vi "update-table-data.vi"(8 "error in (no error)":errorcluster, 9 "valid":bool, 10 "CAN frame":T1 {"payload" format="%x"; "timestamp" format="%<%.7X\n%x>T"; "type" items=["CAN Data"=0, "CAN Remote"=1, "CAN Bus Error"=2, "J1939 Data"=192, "Delay"=224, "Log Trigger"=225, "Start Trigger"=226]; "identifier" format="%x"}, 11 "CANtable in":refnum<class "bAPPdata.lvclass">) -> (0 "error out":errorcluster, 2 "CAN frame out":T1 {"payload" format="%x"; "timestamp" format="%<%.7X\n%x>T"; "type" items=["CAN Data"=0, "CAN Remote"=1, "CAN Bus Error"=2, "J1939 Data"=192, "Delay"=224, "Log Trigger"=225, "Start Trigger"=226]; "identifier" format="%x"}, 3 "CANtable out":refnum<class "bAPPdata.lvclass">)   [LabVIEW 2015, in "bAPPdata.lvclass"]
uses:
  bAPPdata.lvclass
  <vilib>/xnet/xnet.llb/XNET Frame CAN.ctl
  <vilib>/xnet/xnet.llb/XNET Frame Type CAN.ctl
  bAPPdata.lvclass/bAPPdata.ctl
  table-contents.ctl
  subs/frame.type.ctl
  nMsgData.ctl
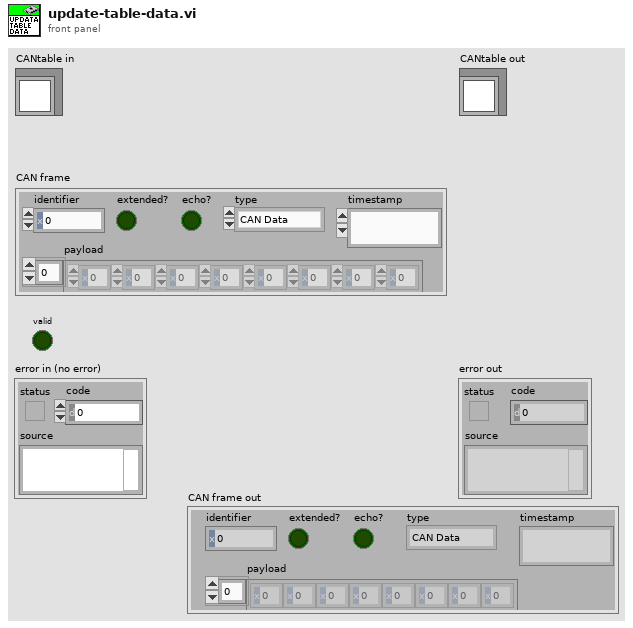
[diagram p1: front panel]
types:
  T1 = typedef "XNET Frame CAN.ctl" = cluster{"timestamp":timestamp, "payload":u8[], "identifier":u32, "type":T2, "extended?":bool, "echo?":bool}
  T2 = typedef "XNET Frame Type CAN.ctl" = u8
  T3 = typedef "nMsgData.ctl" = cluster{"dwID":u32, "count":u32, "dwCycleTime":dbl, "dwTime":dbl, "new msg":bool}
  T4 = typedef "bAPPdata.lvclass/table-contents.ctl" = cluster{"id":u32, "tag":string, "frame.type":T5, "last.frame":T1, "tMsgData":T3, "child.tags":string[], "bit-payload":bool[]}
  T5 = typedef "frame.type.ctl" = enum16{"FRAME NOT DEFINED", "DUT OUTPUT FRAME", "DUT INPUT FRAME"}
  T6 = typedef "bAPPdata.lvclass/table-data.ctl" = T4[]
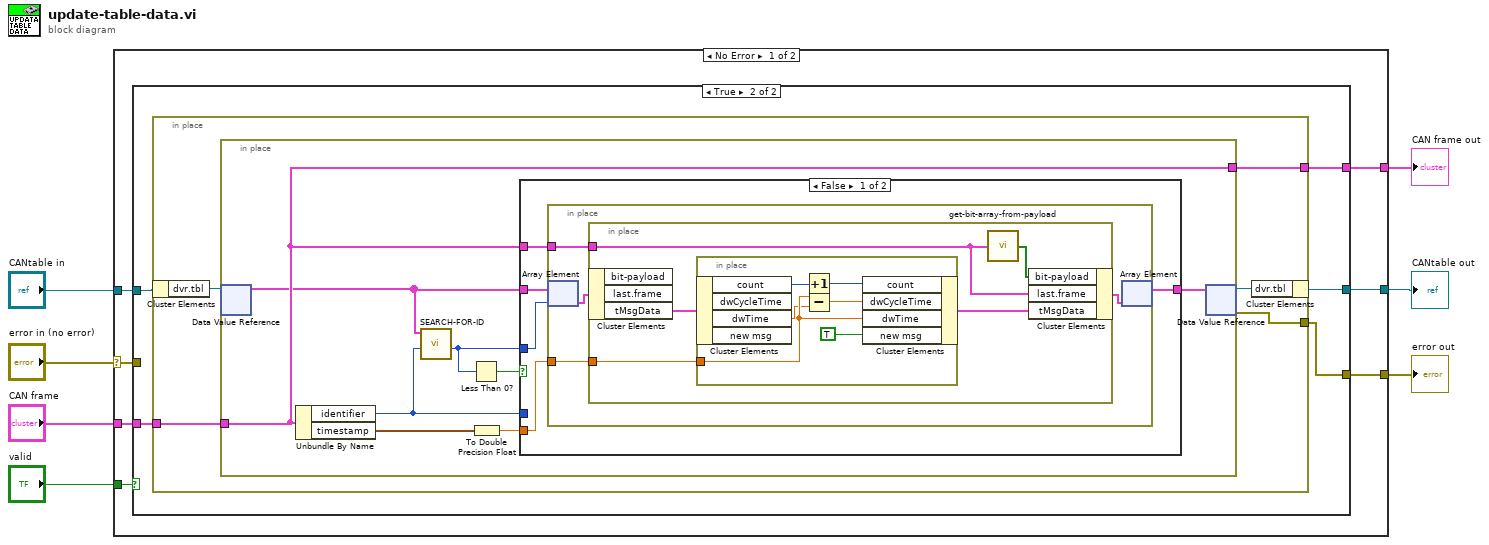
[diagram p0: block diagram]
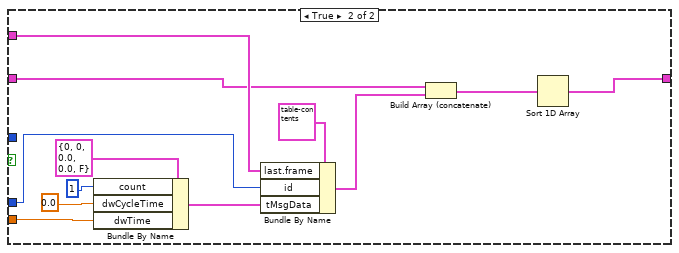
[diagram p3: hidden frame]
diagram:
  n1 = case shown="No Error" "error in (no error)" {
    selector: "error in (no error)" -> [w9 w68]
    tunnel: [w11 w68] -> w6
    tunnel: [w13 w67] -> w4
    tunnel: "CANtable in" -> [w14 w67]
    tunnel: "CAN frame" -> [w12 _]
    tunnel: "valid" -> [w10 _]
    tunnel: [w8 _] -> w1
    frame No Error {
      n2 = case shown="True" w10 {
        tunnel: w14 -> [w16 w21]
        tunnel: [w16 w20] -> w13
        tunnel: w12 -> [_ w19]
        tunnel: [w15 w17] -> w11
        tunnel: w9 -> [w15 _]
        tunnel: [_ w18] -> w8
        frame False {
        }
        frame True {
          n3 = in-place {
            in-place-border: w19 -> [w26]
            in-place-border: [w23] -> w17
            in-place-border: [w22] -> w18
            n4 = in-place-cluster #1(w21) -> ("dvr.tbl"=w25:refnum<data-value>)
            n5 = in-place {
              in-place-border: w26 -> [w34]
              in-place-border: [w34] -> w22
              n6 = in-place-dvr #2(w25) -> (w30:T6)  [unwired: 1 out]
              n7 = Unbundle By Name(w34) -> ("identifier"=w29:u32, "timestamp"=w33:timestamp)
              n8 = call "SEARCH-FOR-ID.vi"("ID"=w29, "tbl.list"=w30) -> ("idx"=w27:i32)  [unwired: 8 in, 1 out]
              n9 = Less Than 0?(x=w27) -> (x < 0?=w31:bool)
              n10 = To Double Precision Float(number=w33) -> (double precision float=w32:dbl)
              n11 = case shown="False" w31 {
                tunnel: w34 -> [w38 w65]
                tunnel: w32 -> [w39 w66]
                tunnel: [w35 w57] -> w28
                tunnel: w29 -> [_ w56]
                tunnel: w30 -> [w37 w55]
                tunnel: w27 -> [w36 _]
                frame False {
                  n12 = in-place {
                    in-place-border: w39 -> [w43]
                    in-place-border: w38 -> [w42]
                    n13 = in-place-array #3(w37, w36) -> (w41:T4)
                    n14 = in-place {
                      in-place-border: w43 -> [w48]
                      in-place-border: w42 -> [w45]
                      n15 = in-place-cluster #4(w41) -> ("tMsgData"=w46:T3)  [unwired: 2 out]
                      n16 = in-place {
                        in-place-border: w48 -> [w52]
                        n17 = in-place-cluster #5(w46) -> ("count"=w50:u32, "dwTime"=w49:dbl)  [unwired: 2 out]
                        n18 = Increment(x=w50) -> (x+1=w54:u32)
                        n19 = Subtract(x=w52, y=w49) -> (x-y=w51:dbl)
                        n20 = in-place-cluster #5("count"=w54, "dwCycleTime"=w51, "dwTime"=w52, "new msg"=TRUE) -> (w47:T3)
                      }
                      n21 = call "get-bit-array-from-payload.vi"("CAN frame"=w45) -> ("Array"=w44:bool[])  [unwired: 4 in]
                      n22 = in-place-cluster #4("bit-payload"=w44, "last.frame"=w45, "tMsgData"=w47) -> (w40:T4)
                    }
                    n23 = in-place-array #3(w40) -> (w35:T6)  [unwired: 1 out]
                  }
                }
                frame True {
                  n24 = Bundle By Name(cluster=T3 {"dwID"=0, "count"=0, "dwCycleTime"=0.0, "dwTime"=0.0, "new msg"=FALSE} ("tMsgData"), "count"=u32 1, "dwCycleTime"=0.0, "dwTime"=w66) -> (w62:T3)
                  n25 = Bundle By Name(cluster=T4 {"id"=0, "tag"="", "frame.type"=enum."FRAME NOT DEFINED", "last.frame"={"timestamp"=timestamp(0 s since 1904-01-01), "payload"=[], "identifier"=0, "type"=0, "extended?"=FALSE, "echo?"=FALSE}, "tMsgData"={"dwID"=0, "count"=0, "dwCycleTime"=0.0, "dwTime"=0.0, "new msg"=FALSE}, "child.tags"=[], "bit-payload"=[]} ("tbl.dta"), "last.frame"=w65, "id"=w56, "tMsgData"=w62) -> (w59:T4)
                  n26 = Build Array (concatenate)(w55, w59) -> (w58:T6)
                  n27 = Sort 1D Array(array=w58) -> (sorted array=w57:T6)
                }
              }
              n28 = in-place-dvr #2(w28) -> (w24:refnum<data-value>, w23:errorcluster)
            }
            n29 = in-place-cluster #1("dvr.tbl"=w24) -> (w20:refnum<class "bAPPdata.lvclass">)
          }
        }
      }
    }
    frame Error {
    }
  }
  "error out" <- w6
  "CANtable out" <- w4
  "CAN frame out" <- w1
